vi "CRYProbe Result.vi"() -> ()   [LabVIEW 2013]
panel:
  out "Source Step":string caption="源步骤"
  in  "Name":string
  in  "Close?":bool
  in  "Update?":bool
  in  "Number":i32
  out "Verdict":bool=TRUE caption="判定"
  out "Unit":string caption="单位"
  out "Limits":string caption="极限"
  out "Tolerance":string caption="公差"
  out "Margin":dbl caption="边缘" format="%#_6p"
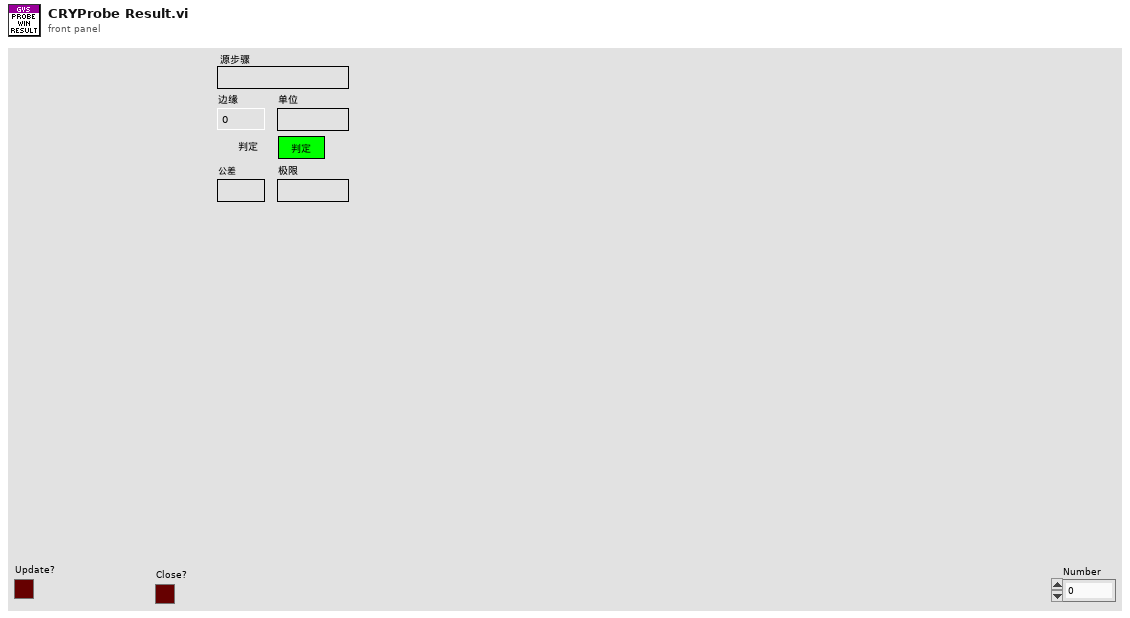
[diagram p1: front panel]
types:
  T1 = typedef "CRYResult Cluster.ctl" = cluster{"Name":string, "Margin":dbl, "unit":string, "Verdict":bool, "Limit":string, "Max/Min":string, "protected":bool, "Step No.":i32, "Test Info":string, "AutoProtect":bool}
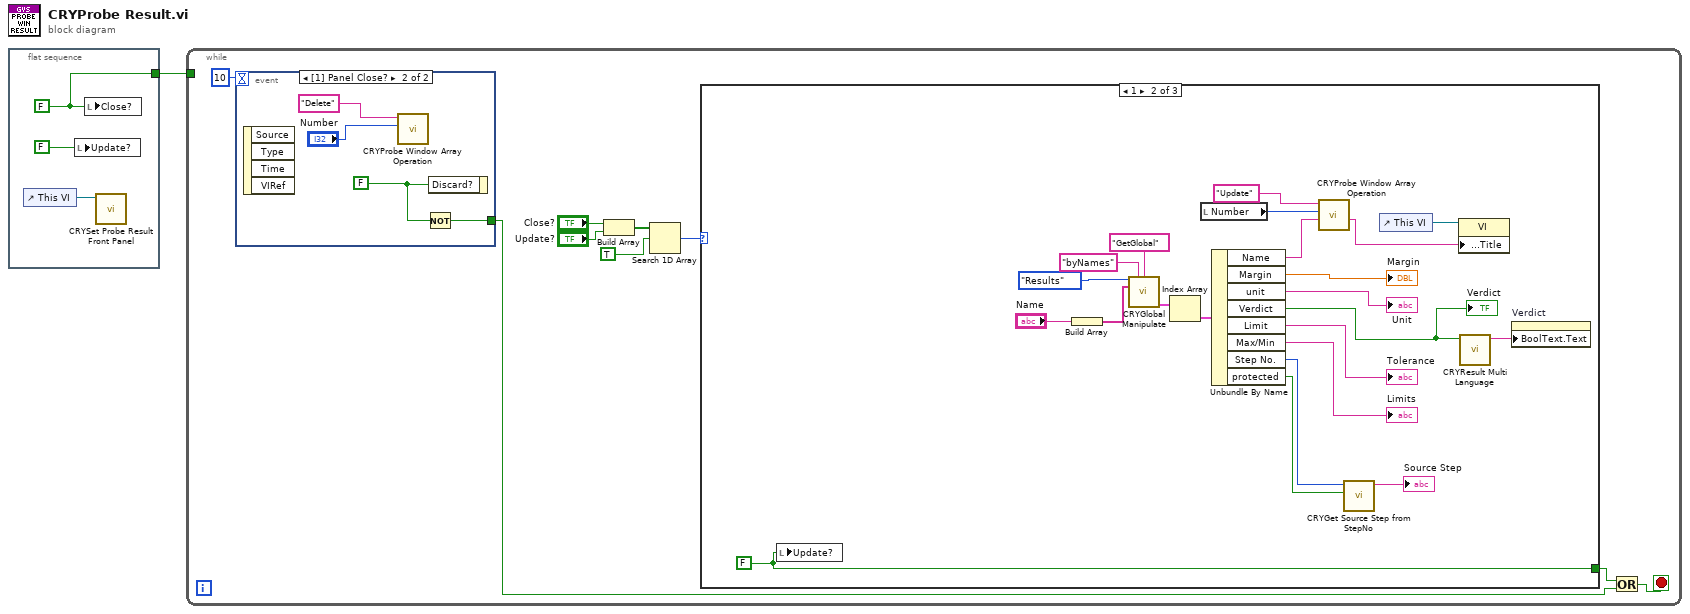
[diagram p0: block diagram]
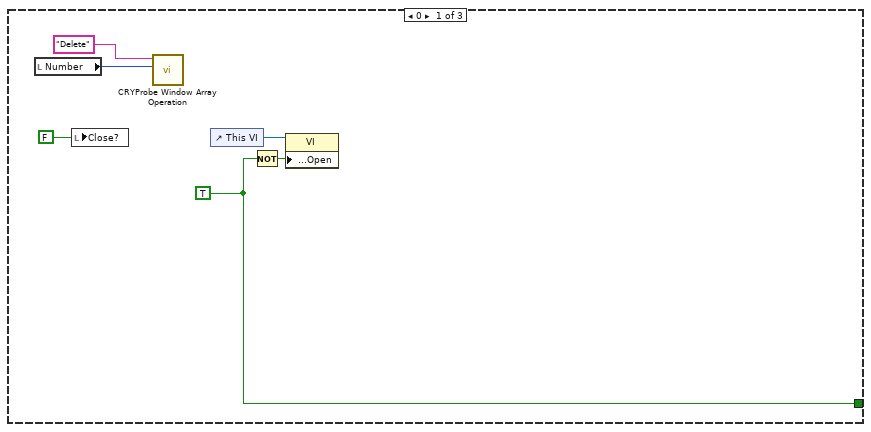
[diagram p2: hidden frame]
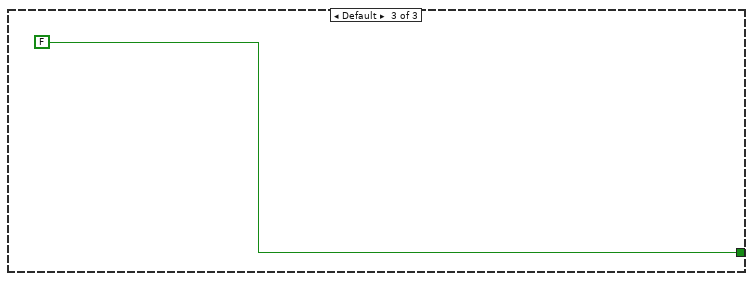
[diagram p3: hidden frame]
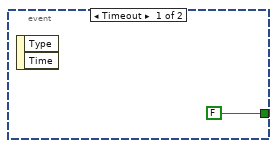
[diagram p4: hidden frame]
diagram:
  n1 = flat-sequence {
    tunnel: [w3] -> w1
    frame #0 {
      w3 = FALSE ("Close?")
      n2 = control-ref of="This VI"() -> (w2:refnum<vi>)
      n3 = local write "Update?"(FALSE ("Close?")) -> ()
      n4 = local write "Close?"(w3) -> ()
      n5 = call "CRYSet Probe Result Front Panel.vi"("Vi Ref"=w2) -> ()  [unwired: 11 in]
    }
  }
  n6 = while {
    tunnel: w1 -> [_]
    stop <- w5 stop-if-true
    n7 = event shown="[1] Panel Close?" {
      selector: _ -> [_ _]
      dyn-events: _ -> [_ _]
      timeout: 10 -> [_ _]
      tunnel: [FALSE ("Discard?") w45] -> w6
      event Timeout {
        n8 = event-data() -> ()  [unwired: 3 out]
      }
      event Panel Close? {
        w46 = FALSE ("Discard?")
        n9 = event-data() -> ()  [unwired: 5 out]
        n10 = call "CRYProbe Window Array Operation.vi"("Number"="Number", "sAction"="Delete") -> ()  [unwired: 1 in, 9 out]
        n11 = Not(x=w46) -> (.not. x?=w45:bool)
        n12 = event-data("Discard?"=w46) -> ()  [unwired: 1 in, 1 out]
      }
    }
    n13 = Build Array("Close?", "Update?") -> (w9:bool[])
    n14 = Search 1D Array(1D array=w9, element=TRUE) -> (index of element=w10:i32)  [unwired: 1 out]
    n15 = case shown="1" w10 {
      tunnel: [w16 w40 FALSE ("Close?")] -> w7
      frame 0 {
        w16 = TRUE ("Discard?")
        n16 = local read "Number"() -> (w15:i32)
        n17 = local write "Close?"(FALSE ("Close?")) -> ()
        n18 = call "CRYProbe Window Array Operation.vi"("Number"=w15, "sAction"="Delete") -> ()  [unwired: 1 in, 9 out]
        n19 = control-ref of="This VI"() -> (w17:refnum<vi>)
        n20 = Not(x=w16) -> (.not. x?=w18:bool)
        n21 = property class="VI"(reference=w17, "Front Panel.Open"=w18) -> ()  [unwired: 1 in, 2 out]
      }
      frame 1 {
        w40 = FALSE ("Close?")
        n22 = local write "Update?"(w40) -> ()
        n23 = Build Array("Name") -> (w20:string[])
        n24 = call "CRYGlobal Manipulate.vi"("Type"=enum16{"Curves", "Values", "Results", "WFM"}."Results" ("Type In"), "sOption"="byNames", "sAction"="GetGlobal", "sData"=w20) -> ("Results Out"=w26:T1[])  [unwired: 5 in, 6 out]
        n25 = Index Array(array=w26) -> (element=w25:T1)  [unwired: 1 in]
        n26 = local read "Number"() -> (w33:i32)
        n27 = Unbundle By Name(w25) -> ("Name"=w34:string, "Margin"=→"Margin":dbl, "unit"=→"Unit":string, "Verdict"=w31:bool, "Limit"=→"Tolerance":string, "Max/Min"=→"Limits":string, "Step No."=w29:i32, "protected"=w28:bool)
        "Verdict" <- w31
        n28 = call "CRYProbe Window Array Operation.vi"("Name"=w34, "Number"=w33, "sAction"="Update") -> ()  [unwired: 9 out]
        n29 = call "CRYGet Source Step from StepNo.vi"("Protect?"=w28, "Step No."=w29) -> ("StepName"=→"Source Step":string)  [unwired: 9 in]
        n30 = control-ref of="This VI"() -> (w35:refnum<vi>)
        n31 = property class="VI"(reference=w35, "Front Panel.Title"=w34) -> ()  [unwired: 1 in, 2 out]
        n32 = call "CRYResult Multi Language.vi"("Verdict"=w31) -> ("ASCII out"=w30:string)  [unwired: 10 in]
        n33 = property on="Verdict" class="Bool (strict)"("BoolText.Text"=w30) -> ()  [unwired: 2 in, 2 out]
      }
      frame Default {
      }
    }
    n34 = Or(x=w7, y=w6) -> (x .or. y?=w5:bool)
  }
